vi "Config NADC Framed Timeslot.vi"(0 "VISA Resource Name":refnum<visa-resource-name>, 1 "Data (0:PN9)":T1(ring), 2 "FIX4 (0000)":i16 format="%.0b", 3 "User File Name (BIN_DATA)":string="BIN_DATA", 5 "Timeslot (1)":i16=1, 7 "Status (T:ON)":bool=TRUE, 9 "Timeslot Type (2:UP TCH)":T2(ring)=enum."UP TCH", 11 "error in (no error)":errorcluster {"code" format="%.0x"}, 12 "SYNC (A91DE4A)":i32=177331786 format="%.0x", 13 "SACCH (000)":i32 format="%.0x", 14 "CDVCC (000)":i32 format="%.0x") -> (4 "VISA Resource Name Out":refnum<visa-resource-name>, 15 "error out":errorcluster {"code" format="%.0x"})   [LabVIEW 2012, in "Agilent ESG Series.lvlib"]
doc: "This VI is used configure a specified Timeslot.\nRun the Config NADC Framed.vi before running this vi.\nRun this vi multiple times to configure multiple Timeslots."
uses:
  Agilent ESG Series.lvlib
panel:
  # "ON"
  # "OFF"
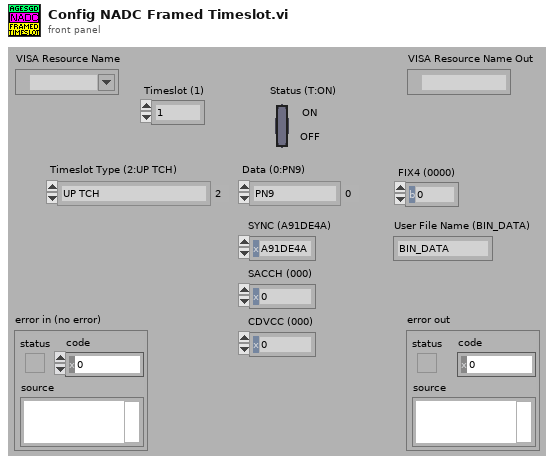
[diagram p1: front panel]
types:
  T1 = enum16{"PN9", "PN15", "FIX4", "USER FILE", "EXT", "4 1's & 4 0's", "8 1's & 8 0's", "16 1's & 16 0's", "32 1's & 32 0's", "64 1's & 64 0's"}
  T2 = enum16{"UP CUSTOM", "DOWN CUSTOM", "UP TCH", "DOWN TCH", "UP TCH ALL", "DOWN TCH ALL"}
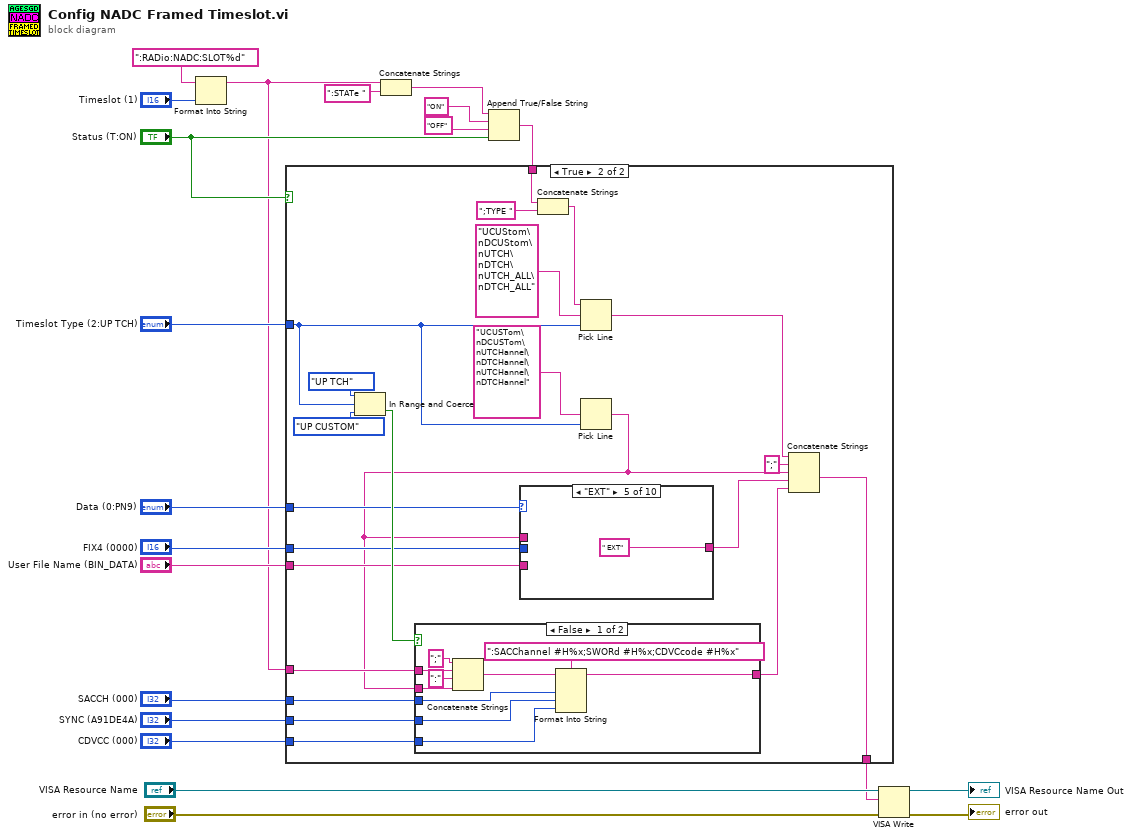
[diagram p0: block diagram]
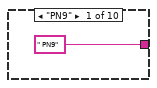
[diagram p3: hidden frame]
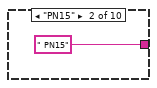
[diagram p4: hidden frame]
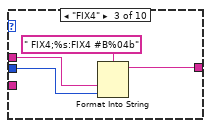
[diagram p5: hidden frame]
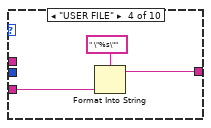
[diagram p6: hidden frame]
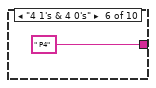
[diagram p7: hidden frame]
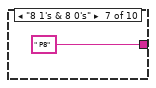
[diagram p8: hidden frame]
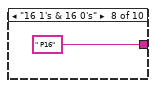
[diagram p9: hidden frame]
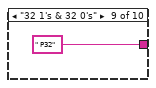
[diagram p10: hidden frame]
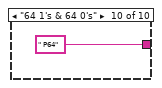
[diagram p11: hidden frame]
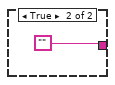
[diagram p12: hidden frame]
diagram:
  n1 = Format Into String(format string=":RADio:NADC:SLOT%d", "Timeslot (1)") -> (resulting string=w2:string)  [unwired: 2 in, 1 out]
  n2 = Concatenate Strings(w2, ":STATe ") -> (w12:string)
  n3 = Append True/False String(1:"Status (T:ON)", 2:"OFF" ("false string"), 3:"ON" ("true string"), 4:w12) -> (0:w11:string)
  n4 = case shown="True" "Status (T:ON)" {
    tunnel: [w22 w43] -> w1
    tunnel: "Timeslot Type (2:UP TCH)" -> [_ w44]
    tunnel: "CDVCC (000)" -> [_ w42]
    tunnel: "SYNC (A91DE4A)" -> [_ w41]
    tunnel: "SACCH (000)" -> [_ w40]
    tunnel: "FIX4 (0000)" -> [_ w34]
    tunnel: "User File Name (BIN_DATA)" -> [_ w33]
    tunnel: "Data (0:PN9)" -> [_ w32]
    tunnel: w11 -> [w22 w31]
    tunnel: w2 -> [_ w26]
    frame False {
    }
    frame True {
      n5 = In Range and Coerce(upper limit=T2."UP TCH" ("hi"), x=w44, lower limit=T2."UP CUSTOM" ("lo")) -> (In Range?=w37:bool)  [unwired: 1 out]
      n6 = Concatenate Strings(w31, ";TYPE ") -> (w29:string)
      n7 = Pick Line(string ("")=w29, multi-line string="UCUStom\nDCUStom\nUTCH\nDTCH\nUTCH_ALL\nDTCH_ALL", line index=w44) -> (output string=w25:string)
      n8 = Pick Line(multi-line string="UCUSTom\nDCUSTom\nUTCHannel\nDTCHannel\nUTCHannel\nDTCHannel", line index=w44) -> (output string=w23:string)  [unwired: 1 in]
      n9 = case shown="False" w37 {
        tunnel: w40 -> [w69 _]
        tunnel: w41 -> [w68 _]
        tunnel: w42 -> [w67 _]
        tunnel: [w65 ""] -> w27
        tunnel: w26 -> [w64 _]
        tunnel: w23 -> [w61 _]
        frame False {
          n10 = Concatenate Strings(";", w64, ":" ("output string"), w61) -> (w63:string)
          n11 = Format Into String(format string=":SACChannel #H%x;SWORd #H%x;CDVCcode #H%x", initial string=w63, w69, w68, w67) -> (resulting string=w65:string)  [unwired: 1 in, 1 out]
        }
        frame True {
        }
      }
      n12 = case shown="\"EXT\"" w32 {
        tunnel: w33 -> [_ _ _ w53 _ _ _ _ _ _]
        tunnel: w34 -> [_ _ w48 _ _ _ _ _ _ _]
        tunnel: [" PN9" " PN15" w49 w51 " EXT" " P4" " P8" " P16" " P32" " P64"] -> w39
        tunnel: w23 -> [_ _ w47 _ _ _ _ _ _ _]
        frame "PN9" {
        }
        frame "PN15" {
        }
        frame "FIX4" {
          n13 = Format Into String(format string=" FIX4;%s:FIX4 #B%04b", w47, w48) -> (resulting string=w49:string)  [unwired: 2 in, 1 out]
        }
        frame "USER FILE" {
          n14 = Format Into String(format string=" \"%s\"", w53) -> (resulting string=w51:string)  [unwired: 2 in, 1 out]
        }
        frame "EXT" {
        }
        frame "4 1's & 4 0's" {
        }
        frame "8 1's & 8 0's" {
        }
        frame "16 1's & 16 0's" {
        }
        frame "32 1's & 32 0's" {
        }
        frame "64 1's & 64 0's" {
        }
      }
      n15 = Concatenate Strings(w25, ";" ("output string"), w23, w39, w27) -> (w43:string)
    }
  }
  n16 = VISA Write(VISA resource name="VISA Resource Name", write buffer=w1, error in (no error)="error in (no error)") -> (VISA resource name out=→"VISA Resource Name Out":refnum<visa-resource-name>, error out=→"error out":errorcluster)  [unwired: 1 out]
